vi "Read Child Class Info.vi"(8 "error in (no error)":errorcluster) -> (0 "error out":errorcluster, 1 "Class Names":string[](array[string]), 2 "Library Versions":T1(array[cluster]), 3 "Private Data Clusters":variant[](array[variant]))   [LabVIEW 2017, in "TestLibrary.lvlib"]
uses:
  TestLibrary.lvlib
  Composition/Composition.lvlib
  ChildClass/ChildClass.lvclass
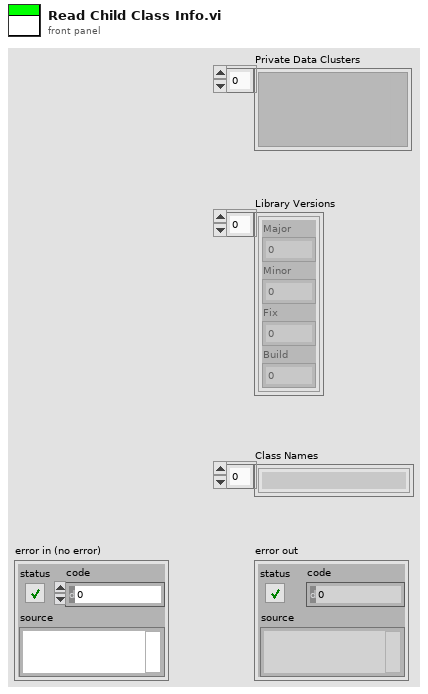
[diagram p1: front panel]
types:
  T1 = cluster{"Major":u16, "Minor":u16, "Fix":u16, "Build":u16}[]
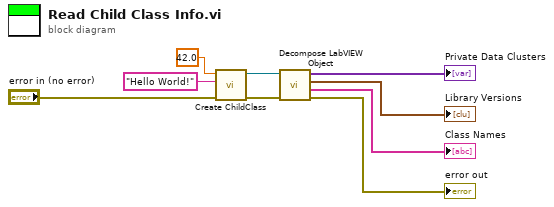
[diagram p0: block diagram]
diagram:
  n1 = call "Create ChildClass.vi"("error in (no error)"="error in (no error)", "String"="Hello World!", "Numeric"=42.0) -> ("error out"=w8:errorcluster, "ChildClass"=w9:refnum<class "ChildClass.lvclass">)  [unwired: 7 in]
  n2 = call "Decompose LabVIEW Object.vi"("error in (no error)"=w8, "LabVIEW Object"=w9) -> ("error out"=→"error out":errorcluster, "Class Names"=→"Class Names":string[], "Library Versions"=→"Library Versions":T1, "Private Data Clusters"=→"Private Data Clusters":variant[])  [unwired: 6 in]
